vi "segmentgraph.vi"(8 "error in (no error)":errorcluster, 10 "Y":dbl[](array[numeric])=[0.0, 0.06279051952931337, 0.12533323356430426, 0.1873813145857246, 0.2486898871648548, 0.3090169943749474, 0.3681245526846779, 0.4257792915650727, 0.4817536741017153, 0.5358267949789967, 0.5877852522924731, 0.6374239897486896, 0.6845471059286886, 0.7289686274214116, 0.7705132427757893, 0.8090169943749475, 0.8443279255020151, 0.8763066800438637, 0.9048270524660196, 0.9297764858882513, 0.9510565162951535, 0.9685831611286311, 0.9822872507286886, 0.9921147013144779, 0.9980267284282716, 1.0, 0.9980267284282716, 0.9921147013144778, 0.9822872507286886, 0.9685831611286312, 0.9510565162951536, 0.9297764858882513, 0.9048270524660195, 0.8763066800438635, 0.844327925502015, 0.8090169943749475, 0.7705132427757893, 0.7289686274214114, 0.6845471059286888, 0.6374239897486899, 0.5877852522924732, 0.535826794978997, 0.4817536741017156, 0.4257792915650729, 0.36812455268467814, 0.3090169943749475, 0.24868988716485482, 0.18738131458572502, 0.12533323356430454, 0.06279051952931358, 1.2246467991473532e-16, -0.06279051952931335, -0.12533323356430429, -0.18738131458572477, -0.24868988716485502, -0.30901699437494773, -0.3681245526846783, -0.42577929156507227, -0.481753674101715, -0.5358267949789964, -0.587785252292473, -0.6374239897486896, -0.6845471059286887, -0.7289686274214113, -0.7705132427757894, -0.8090169943749473, -0.8443279255020153, -0.8763066800438636, -0.9048270524660198, -0.9297764858882511, -0.9510565162951535, -0.968583161128631, -0.9822872507286887, -0.9921147013144778, -0.9980267284282716, -1.0, -0.9980267284282716, -0.9921147013144779, -0.9822872507286887, -0.9685831611286311, -0.9510565162951536, -0.9297764858882512, -0.9048270524660199, -0.8763066800438638, -0.8443279255020155, -0.8090169943749476, -0.7705132427757896, -0.7289686274214116, -0.684547105928689, -0.6374239897486896, -0.5877852522924734, -0.5358267949789963, -0.4817536741017153, -0.4257792915650722, -0.3681245526846787, -0.3090169943749476, -0.24868988716485535, -0.18738131458572468, -0.12533323356430465, -0.06279051952931326], 11 "X":dbl[](array[numeric])=[1.0, 0.9980267284282716, 0.9921147013144779, 0.9822872507286887, 0.9685831611286311, 0.9510565162951535, 0.9297764858882515, 0.9048270524660195, 0.8763066800438636, 0.8443279255020151, 0.8090169943749475, 0.7705132427757893, 0.7289686274214116, 0.6845471059286886, 0.6374239897486896, 0.5877852522924731, 0.5358267949789965, 0.48175367410171516, 0.42577929156507266, 0.3681245526846781, 0.30901699437494745, 0.24868988716485496, 0.18738131458572474, 0.12533323356430426, 0.06279051952931353, 6.123233995736766e-17, -0.0627905195293134, -0.12533323356430437, -0.18738131458572482, -0.24868988716485463, -0.30901699437494734, -0.368124552684678, -0.4257792915650727, -0.48175367410171543, -0.5358267949789969, -0.587785252292473, -0.6374239897486897, -0.6845471059286887, -0.7289686274214113, -0.7705132427757891, -0.8090169943749473, -0.8443279255020149, -0.8763066800438634, -0.9048270524660194, -0.9297764858882513, -0.9510565162951535, -0.9685831611286311, -0.9822872507286886, -0.9921147013144778, -0.9980267284282716, -1.0, -0.9980267284282716, -0.9921147013144779, -0.9822872507286886, -0.9685831611286311, -0.9510565162951535, -0.9297764858882512, -0.9048270524660197, -0.8763066800438637, -0.8443279255020152, -0.8090169943749476, -0.7705132427757893, -0.7289686274214116, -0.684547105928689, -0.6374239897486895, -0.5877852522924732, -0.5358267949789963, -0.48175367410171527, -0.42577929156507216, -0.3681245526846786, -0.30901699437494756, -0.2486898871648553, -0.18738131458572463, -0.1253332335643046, -0.06279051952931321, -1.8369701987210297e-16, 0.06279051952931283, 0.12533323356430423, 0.18738131458572427, 0.24868988716485493, 0.30901699437494723, 0.36812455268467825, 0.4257792915650718, 0.48175367410171493, 0.535826794978996, 0.5877852522924729, 0.6374239897486893, 0.6845471059286886, 0.7289686274214112, 0.7705132427757894, 0.8090169943749473, 0.8443279255020153, 0.8763066800438636, 0.9048270524660197, 0.9297764858882511, 0.9510565162951535, 0.968583161128631, 0.9822872507286887, 0.9921147013144778, 0.9980267284282716]) -> (0 "error out":errorcluster, 1 "y out":dbl[](array[numeric]), 2 "xout":dbl[](array[numeric]), 3 "Segment":cluster{dbl[], dbl[]})   [LabVIEW 2016]
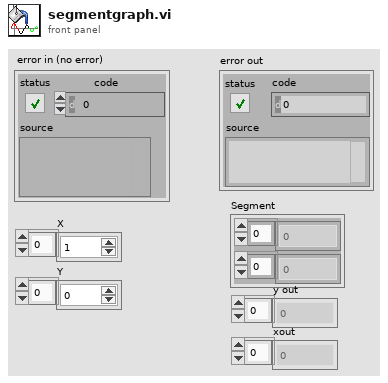
[diagram p1: front panel]
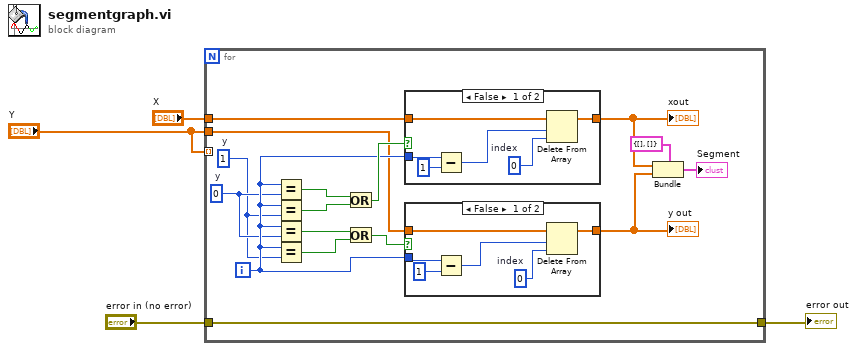
[diagram p0: block diagram]
diagram:
  n1 = for {
    tunnel: "Y" -> [_] mode=indexing
    tunnel: "Y" -> [w6]
    tunnel: "X" -> [w5]
    tunnel: "error in (no error)" -> [w8]
    tunnel: [w8] -> w1
    i -> [w11]
    w9 = 1  # y
    w10 = 0  # y
    n2 = Equal?(x=w11, y=w10) -> (x = y?=w16:bool)
    n3 = Equal?(x=w11, y=w9) -> (x = y?=w17:bool)
    n4 = Equal?(x=w11, y=w10) -> (x = y?=w13:bool)
    n5 = Equal?(x=w11, y=w9) -> (x = y?=w12:bool)
    n6 = Or(x=w16, y=w17) -> (x .or. y?=w15:bool)
    n7 = Or(x=w13, y=w12) -> (x .or. y?=w14:bool)
    n8 = case shown="False" w15 {
      tunnel: w5 -> [w33 w34]
      tunnel: [w31 w34] -> w18
      tunnel: w11 -> [w30 _]
      frame False {
        w32 = 0  # index
        n9 = Subtract(x=w30, y=1) -> (x-y=w28:i32)
        n10 = Delete From Array(array=w33, length=w28, index=w32) -> (array with subset deleted=w31:dbl[])  [unwired: 1 out]
      }
      frame True {
      }
    }
    "xout" <- w18
    n11 = case shown="False" w14 {
      tunnel: w6 -> [w26 w27]
      tunnel: [w21 w27] -> w7
      tunnel: w11 -> [w24 _]
      frame False {
        w25 = 0  # index
        n12 = Subtract(x=w24, y=1) -> (x-y=w22:i32)
        n13 = Delete From Array(array=w26, length=w22, index=w25) -> (array with subset deleted=w21:dbl[])  [unwired: 1 out]
      }
      frame True {
      }
    }
    "y out" <- w7
    n14 = Bundle(cluster=cluster{dbl[], dbl[]} {[], []}, w18, w7) -> (→"Segment":cluster{dbl[], dbl[]})
  }
  "error out" <- w1
